vi "Test UI Manager API.vi"() -> ()   [LabVIEW 2022 SP3]
doc: "UI Manager API Tester.\n\n<b>Note:</b> This VI was modified by the <b>Validate DQMH Module</b> tool to add the 'Show Main VI Diagram on Init' functionality included in DQMH 6.1.\n\n<b>Note:</b> This VI was modified by the <b>Validate DQMH Module</b> tool to upgrade its Error Reported event frame to use an improved mechanism for displaying error information.\n\n____\nHAMPEL SOFTWARE ENGINEERING v2.6.0 (2023-12-19 10:54)"
uses:
  <vilib>/Utility/error.llb/DialogType.ctl
  <vilib>/Hampel Software Engineering/HSE Logger/LogRecord/LogRecord.lvclass/LogRecord.ctl
  UI Manager.lvlib
  Libraries/hse-libraries/Source/hse-dqmh/hse-dqmh.lvlib
  <vilib>/Hampel Software Engineering/HSE Logger/LogRecord/LogRecord.lvclass
  <vilib>/Hampel Software Engineering/HSE Logger/hse-logger.lvlib
panel:
  out "User Level":string
  out "User Name":string
  in  "Get User Level":bool
  in  "External Login":bool
  in  "Show Main VI Diagram on Init (F)":bool
  out "CLI Arguments out":string[](array[string])
  in  "Get CLI Arguments":bool
  in  "CLI Arguments in":string[](array[string])
  in  "Set CLI Arguments":bool
  in  "Remove Module from Run-Time Menu":bool
  in  "Descriptor":string
  in  "Shutdown Application":bool
  in  "Closeable?":bool
  in  "Set Window Closeable State":bool
  in  "Visible?":bool
  in  "Set Run-Time Menu Visibility":bool
  in  "Add Modules":bool
  in  "Modules Path":path
  in  "Add Mod to Menu":bool
  in  "Module DQMH Path":path
  in  "Btn_SystemMessage":bool
  in  "Prepare":bool
  in  "Configure":bool
  in  "Show PROJECT-ABOUT":bool
  in  "Show HSE-ABOUT":bool
  in  "Load RT Menu":bool
  in  "Run-Time Menu Path":path
  in  "Show Block Diagram":bool
  in  "Stop Module":bool
  in  "Start Module":bool
  in  "Hide Module Panel":bool
  in  "Show Module Panel":bool
  out "Status":string
  out "Module Running?":bool
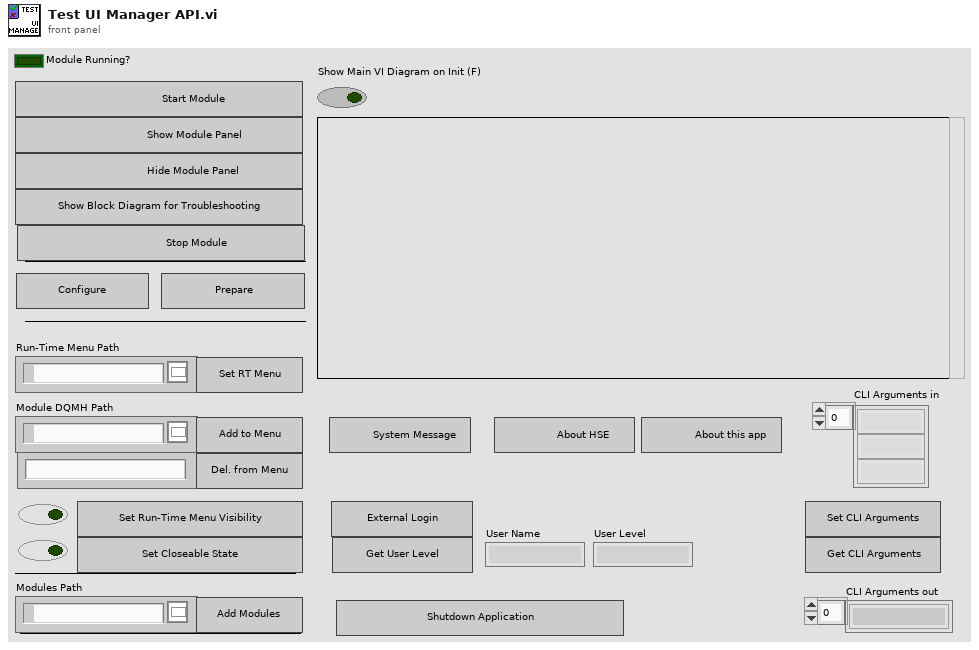
[diagram p1: front panel]
types:
  T1 = typedef "UI Manager.lvlib/Broadcast Events--cluster.ctl" = cluster{"Module Did Init":refnum<user-event>, "Status Updated":refnum<user-event>, "Error Reported":refnum<user-event>, "Module Did Stop":refnum<user-event>, "Update Module Execution Status":refnum<user-event>, "System Message":refnum<user-event>, "Login":refnum<user-event>, "Key down":refnum<user-event>}
  T2 = typedef "DialogType.ctl" = u16
  T3 = typedef "hse-dqmh.lvlib/System Message Source.ctl" = enum16{"module", "application", "network"}
  T4 = typedef "hse-logger.lvlib/LogLevel.ctl" = enum16{"DEBUG", "INFO", "WARNING", "ERROR", "CRITICAL"}
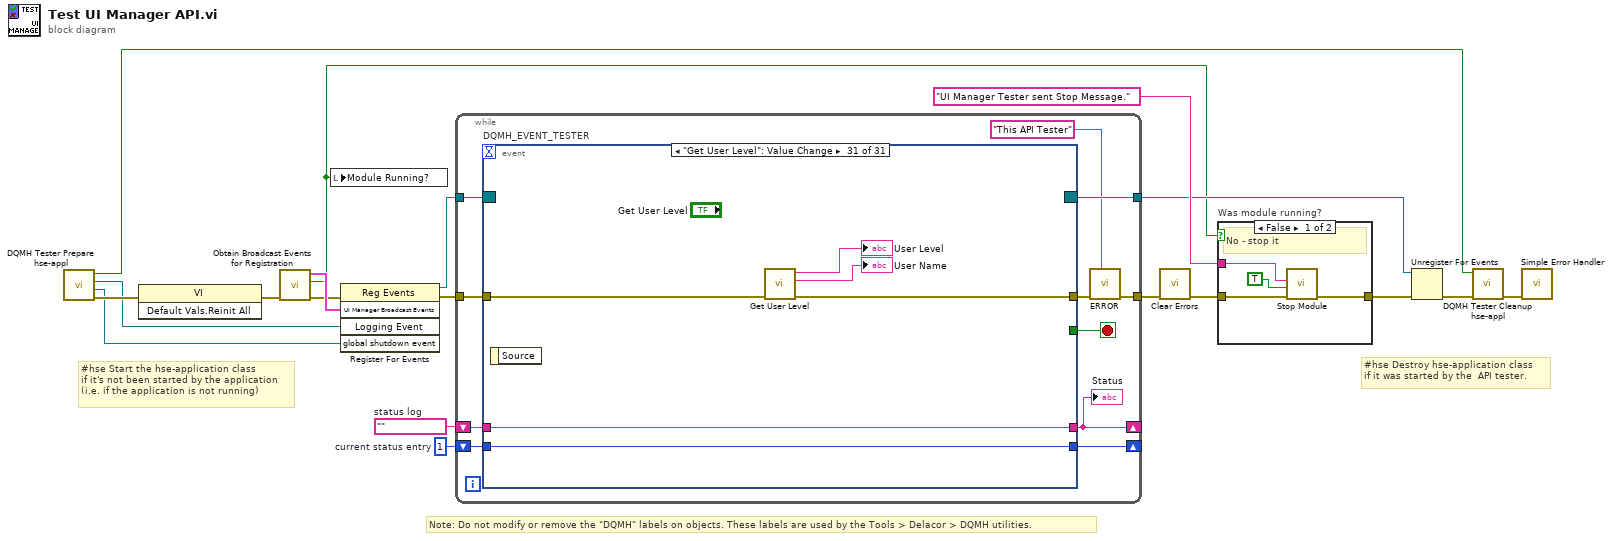
[diagram p0: block diagram]
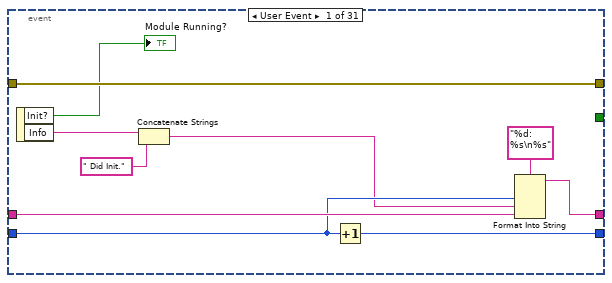
[diagram p3: hidden frame]
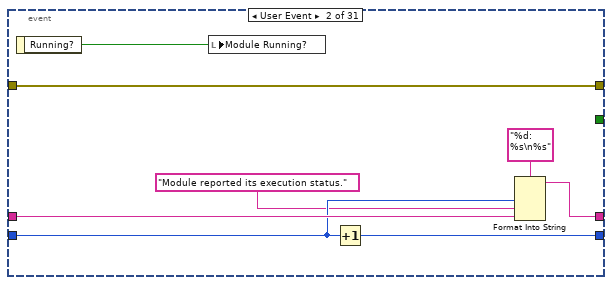
[diagram p4: hidden frame]
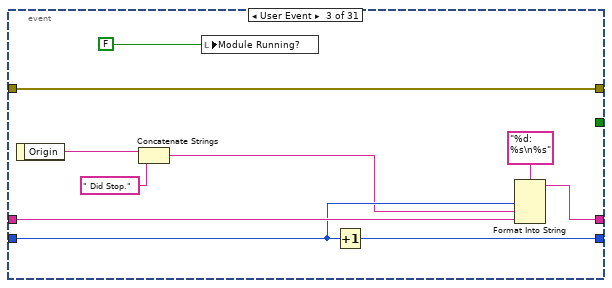
[diagram p5: hidden frame]
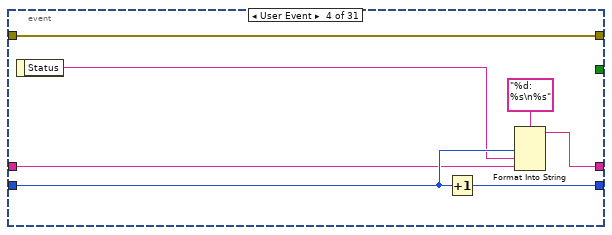
[diagram p6: hidden frame]
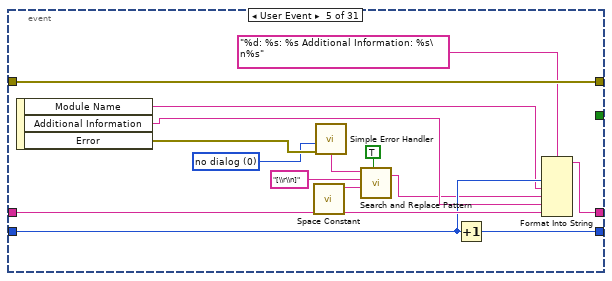
[diagram p7: hidden frame]
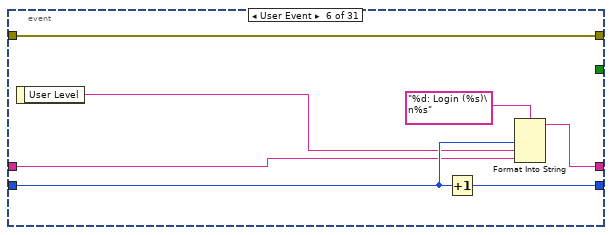
[diagram p8: hidden frame]
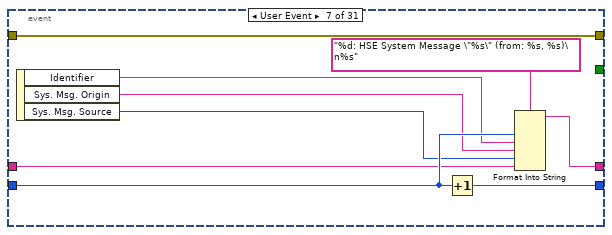
[diagram p9: hidden frame]
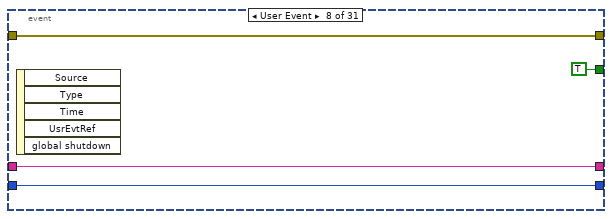
[diagram p10: hidden frame]
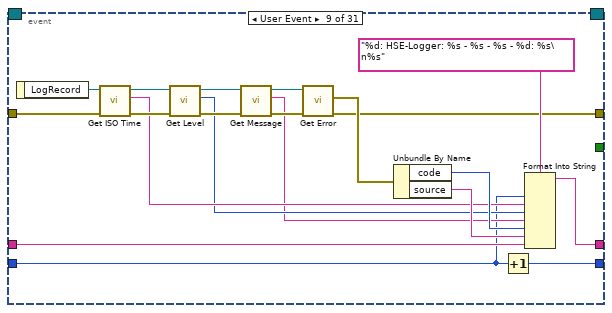
[diagram p11: hidden frame]
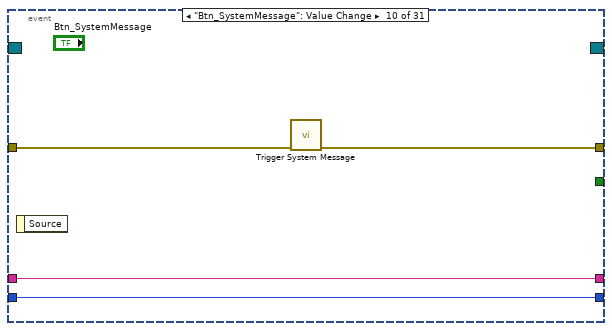
[diagram p12: hidden frame]
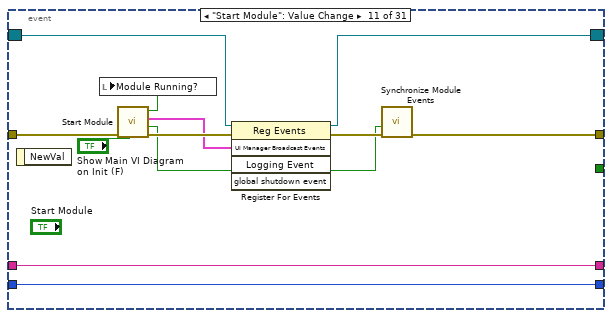
[diagram p13: hidden frame]
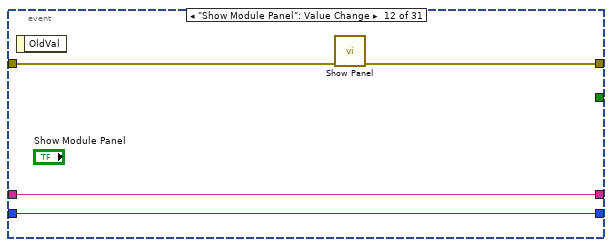
[diagram p14: hidden frame]
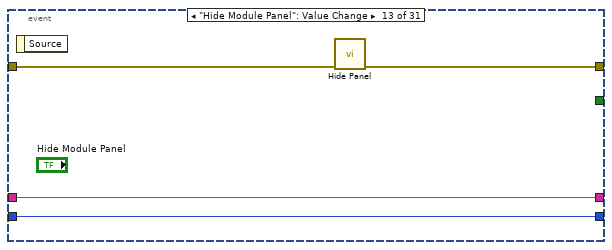
[diagram p15: hidden frame]
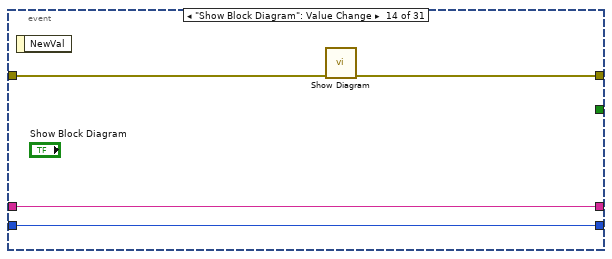
[diagram p16: hidden frame]
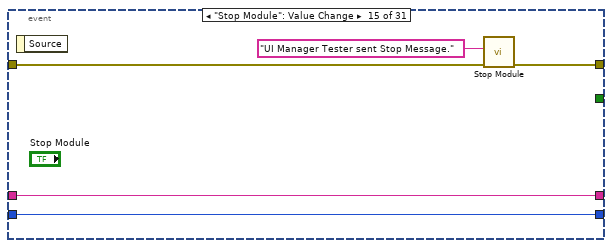
[diagram p17: hidden frame]
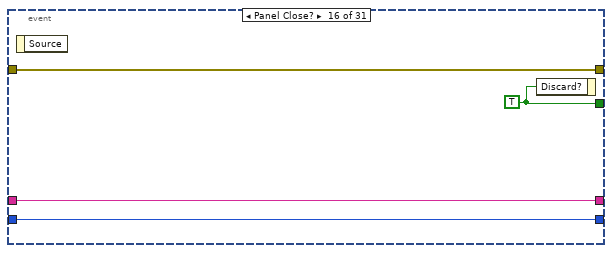
[diagram p18: hidden frame]
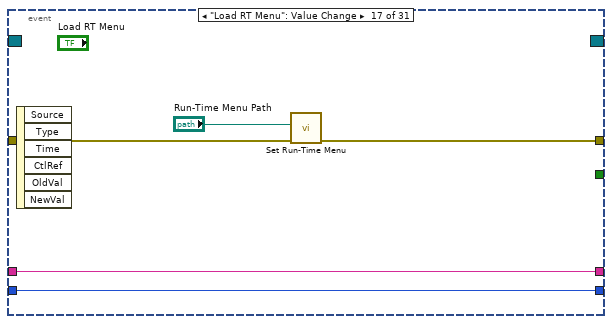
[diagram p19: hidden frame]
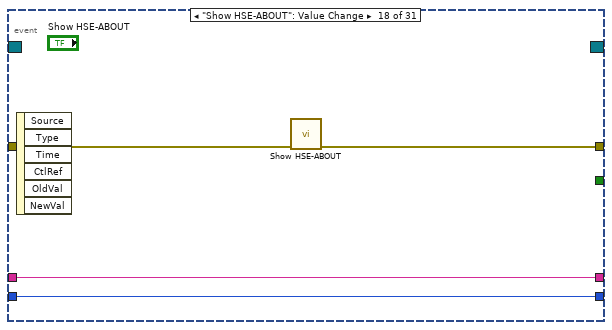
[diagram p20: hidden frame]
diagram:
  w16 = 1  # current status entry
  w17 = ""  # status log
  # "#hse Start the hse-application class \nif it's not been started by the application\n(i.e. if the application is not running)"
  # "#hse Destroy hse-application class \nif it was started by the  API tester."
  # "Note: Do not modify or remove the \"DQMH\" labels on objects. These labels are used by the Tools > Delacor > DQMH utilities."
  n1 = call "DQMH Tester Prepare hse-appl.vi"() -> ("error out"=w9:errorcluster, "global shutdown event"=w1:refnum<user-event>, "Logging Event"=w6:refnum<user-event>, "Started?"=w5:bool)  [unwired: 8 in]
  n2 = invoke class="VI" method="Default Vals.Reinit All"(error in=w9) -> (error out=w8:errorcluster)  [unwired: 2 in, 2 out]
  n3 = call "Obtain Broadcast Events for Registration.vi"("error in (no error)"=w8) -> ("error out"=w7:errorcluster, "Already running?"=w4:bool, "UI Manager Broadcast Events"=w14:T1)  [unwired: 8 in]
  n4 = local write "Module Running?"(w4) -> ()
  n5 = register-events(error in=w7, w14, w6, w1) -> (reference out=w13:refnum<event-registration>, error out=w15:errorcluster)  [unwired: 1 in]
  n6 = while {
    tunnel: w13 -> [w30]
    tunnel: [w21] -> w3
    shift-right: [w26] -> _
    shift-left: w17 -> [w28]
    shift-right: [w27] -> _
    shift-left: w16 -> [w29]
    tunnel: w15 -> [w25]
    tunnel: [w24] -> w12
    stop <- w22 stop-if-true
    n7 = event "DQMH_EVENT_TESTER" shown="[30] \"Get User Level\": Value Change" {
      selector: w30 -> [_ _ _ _ _ _ _ _ _ _ w129 _ _ _ _ _ _ _ _ _ _ _ _ _ _ _ _ _ _ _ _]
      dyn-events: [_ _ _ _ _ _ _ _ _ _ w128 _ _ _ _ _ _ _ _ _ _ _ _ _ _ _ _ _ _ _ _] -> w24
      timeout: _ -> [_ _ _ _ _ _ _ _ _ _ _ _ _ _ _ _ _ _ _ _ _ _ _ _ _ _ _ _ _ _ _]
      tunnel: [_ _ _ _ _ _ _ TRUE ("Discard?") _ _ _ _ _ _ _ w156 _ _ _ _ _ _ _ _ _ _ _ _ _ _ _] -> w22
      tunnel: [w40 w42 w49 w59 w80 w87 w95 w99 w102 w120 w127 w139 w143 w144 w150 w153 w158 w162 w166 w170 w174 w180 w186 w191 w196 w201 w206 w211 w216 w222 w228] -> w23
      tunnel: w29 -> [w36 w46 w56 w62 w77 w85 w93 w97 w103 w121 w132 w137 w141 w145 w151 w154 w159 w163 w167 w171 w175 w181 w187 w192 w197 w202 w207 w212 w217 w223 w229]
      tunnel: w28 -> [w37 w47 w57 w61 w79 w82 w89 w98 w104 w122 w133 w138 w142 w146 w152 w155 w160 w164 w168 w172 w176 w182 w188 w193 w198 w203 w208 w213 w218 w224 w230]
      tunnel: [w34 w44 w54 w63 w78 w83 w92 w98 w100 w122 w133 w138 w142 w146 w152 w155 w160 w164 w168 w172 w176 w182 w188 w193 w198 w203 w208 w213 w218 w224 w230] -> w26
      tunnel: [w35 w45 w55 w65 w76 w84 w93 w97 w101 w121 w132 w137 w141 w145 w151 w154 w159 w163 w167 w171 w175 w181 w187 w192 w197 w202 w207 w212 w217 w223 w229] -> w27
      tunnel: w25 -> [w40 w42 w49 w59 w80 w87 w95 w99 w105 w123 w126 w136 w140 w147 w148 w153 w161 w165 w169 w173 w177 w183 w189 w194 w199 w204 w209 w214 w219 w225 w231]
      event User Event {
        n8 = event-data() -> ("Init?"=→"Module Running?":bool, "Info"=w33:string)  [unwired: 1 in]
        n9 = Concatenate Strings(w33, " Did Init.") -> (w32:string)
        n10 = Increment(x=w36) -> (x+1=w35:i32)
        n11 = Format Into String(format string="%d: %s\n%s", w36, w32, w37) -> (resulting string=w34:string)  [unwired: 2 in, 1 out]
      }
      event User Event {
        n12 = event-data() -> ("Running?"=w41:bool)  [unwired: 1 in]
        n13 = local write "Module Running?"(w41) -> ()
        n14 = Increment(x=w46) -> (x+1=w45:i32)
        n15 = Format Into String(format string="%d: %s\n%s", w46, "Module reported its execution status.", w47) -> (resulting string=w44:string)  [unwired: 2 in, 1 out]
      }
      event User Event {
        n16 = event-data() -> ("Origin"=w53:string)  [unwired: 1 in]
        n17 = Concatenate Strings(w53, " Did Stop.") -> (w52:string)
        n18 = local write "Module Running?"(FALSE ("Module Did Init?")) -> ()
        n19 = Increment(x=w56) -> (x+1=w55:i32)
        n20 = Format Into String(format string="%d: %s\n%s", w56, w52, w57) -> (resulting string=w54:string)  [unwired: 2 in, 1 out]
      }
      event User Event {
        n21 = event-data() -> ("Status"=w60:string)  [unwired: 1 in]
        n22 = Increment(x=w62) -> (x+1=w65:i32)
        n23 = Format Into String(format string="%d: %s\n%s", w62, w60, w61) -> (resulting string=w63:string)  [unwired: 2 in, 1 out]
      }
      event User Event {
        w72 = T2 0 items=["no dialog", "OK message", "continue or stop message", "OK message + warnings", "continue/stop + warnings"] ("type of dialog (OK msg:1)")
        n24 = event-data() -> ("Module Name"=w73:string, "Additional Information"=w74:string, "Error"=w75:errorcluster)  [unwired: 1 in]
        n25 = call <vilib>:"Space Constant.vi"() -> ("String"=w68:string)
        n26 = call <vilib>:"Simple Error Handler.vi"("type of dialog (OK msg:1)"=w72, "error in (no error)"=w75) -> ("message"=w71:string)  [unwired: 3 in, 4 out]
        n27 = call <vilib>:"Search and Replace Pattern.vi"("string"=w71, "regular expression (\"\")"="[\\r\\n]" ("regular expression (\"\")"), "replace string (\"\")"=w68, "replace all? (F)"=TRUE ("replace all CR/LF with spaces")) -> ("result string"=w70:string)  [unwired: 1 in, 1 out]
        n28 = Increment(x=w77) -> (x+1=w76:i32)
        n29 = Format Into String(format string="%d: %s: %s Additional Information: %s\n%s", w77, w73, w70, w74, w79) -> (resulting string=w78:string)  [unwired: 2 in, 1 out]
      }
      event User Event {
        n30 = event-data() -> ("User Level"=w81:string)  [unwired: 1 in]
        n31 = Increment(x=w85) -> (x+1=w84:i32)
        n32 = Format Into String(format string="%d: Login (%s)\n%s", w85, w81, w82) -> (resulting string=w83:string)  [unwired: 2 in, 1 out]
      }
      event User Event {
        n33 = event-data() -> ("Identifier"=w91:string, "Sys. Msg. Origin"=w90:string, "Sys. Msg. Source"=w88:T3)  [unwired: 1 in]
        n34 = Increment(x=w93) -> ()  [unwired: 1 out]
        n35 = Format Into String(format string="%d: HSE System Message \"%s\" (from: %s, %s)\n%s", w93, w91, w90, w88, w89) -> (resulting string=w92:string)  [unwired: 2 in, 1 out]
      }
      event User Event {
        n36 = event-data() -> ()  [unwired: 1 in, 5 out]
      }
      event User Event {
        n37 = event-data() -> ("LogRecord"=w106:refnum<class "LogRecord.lvclass">)  [unwired: 1 in]
        n38 = call <vilib>:"Get ISO Time.vi"("error in"=w105, "LogRecord in"=w106) -> ("error out"=w119:errorcluster, "ISO Time"=w109:string, "LogRecord out"=w118:refnum<class "LogRecord.lvclass">)  [unwired: 7 in]
        n39 = call <vilib>:"Get Level.vi"("error in"=w119, "LogRecord in"=w118) -> ("error out"=w116:errorcluster, "Level"=w108:T4, "LogRecord out"=w117:refnum<class "LogRecord.lvclass">)  [unwired: 7 in]
        n40 = call <vilib>:"Get Message.vi"("error in"=w116, "LogRecord in"=w117) -> ("error out"=w114:errorcluster, "Message"=w107:string, "LogRecord out"=w115:refnum<class "LogRecord.lvclass">)  [unwired: 7 in]
        n41 = call <vilib>:"Get Error.vi"("error in"=w114, "LogRecord in"=w115) -> ("error out"=w102:errorcluster, "Error"=w110:errorcluster)  [unwired: 7 in, 1 out]
        n42 = Unbundle By Name(w110) -> ("code"=w112:i32, "source"=w111:string)
        n43 = Increment(x=w103) -> (x+1=w101:i32)
        n44 = Format Into String(format string="%d: HSE-Logger: %s - %s - %s - %d: %s\n%s", w103, w109, w108, w107, w112, w111, w104) -> (resulting string=w100:string)  [unwired: 2 in, 1 out]
      }
      event "Btn_SystemMessage": Value Change {
        n45 = event-data() -> ()  [unwired: 1 in, 1 out]
        n46 = call "Trigger System Message.vi"("error in (no error)"=w123) -> ("error out"=w120:errorcluster)  [unwired: 10 in]
      }
      event "Start Module": Value Change {
        n47 = event-data() -> ()  [unwired: 1 in, 1 out]
        n48 = call "Start Module.vi"("Show Main VI Diagram on Init (F)"="Show Main VI Diagram on Init (F)", "error in (no error)"=w126) -> ("error out"=w134:errorcluster, "Wait for Event Sync?"=w131:bool, "UI Manager Broadcast Events"=w130:T1, "Module Was Already Running?"=w125:bool)  [unwired: 6 in]
        n49 = local write "Module Running?"(w125) -> ()
        n50 = register-events(reference=w129, error in=w134, w130) -> (reference out=w128:refnum<event-registration>, error out=w135:errorcluster)  [unwired: 2 in]
        n51 = call "Synchronize Module Events.vi"("error in (no error)"=w135, "Wait for Event Sync?"=w131) -> ("error out"=w127:errorcluster)  [unwired: 9 in]
      }
      event "Show Module Panel": Value Change {
        n52 = event-data() -> ()  [unwired: 1 in, 1 out]
        n53 = call "Show Panel.vi"("error in (no error)"=w136) -> ("error out"=w139:errorcluster)  [unwired: 10 in]
      }
      event "Hide Module Panel": Value Change {
        n54 = event-data() -> ()  [unwired: 1 in, 1 out]
        n55 = call "Hide Panel.vi"("error in (no error)"=w140) -> ("error out"=w143:errorcluster)  [unwired: 10 in]
      }
      event "Show Block Diagram": Value Change {
        n56 = event-data() -> ()  [unwired: 1 in, 1 out]
        n57 = call "Show Diagram.vi"("error in (no error)"=w147) -> ("error out"=w144:errorcluster)  [unwired: 10 in]
      }
      event "Stop Module": Value Change {
        n58 = event-data() -> ()  [unwired: 1 in, 1 out]
        n59 = call "Stop Module.vi"("error in (no error)"=w148, "Origin"="UI Manager Tester sent Stop Message.") -> ("error out"=w150:errorcluster)  [unwired: 9 in]
      }
      event Panel Close? {
        w156 = TRUE ("Discard?")
        n60 = event-data() -> ()  [unwired: 1 in, 1 out]
        n61 = event-data("Discard?"=w156) -> ()  [unwired: 1 in, 1 out]
      }
      event "Load RT Menu": Value Change {
        n62 = event-data() -> ()  [unwired: 1 in, 6 out]
        n63 = call "Set Run-Time Menu.vi"("error in (no error)"=w161, "Run-Time Menu Path"="Run-Time Menu Path") -> ("error out"=w158:errorcluster)  [unwired: 9 in]
      }
      event "Show HSE-ABOUT": Value Change {
        n64 = event-data() -> ()  [unwired: 1 in, 6 out]
        n65 = call "Show HSE-ABOUT.vi"("error in (no error)"=w165) -> ("error out"=w162:errorcluster)  [unwired: 10 in]
      }
      event "Show PROJECT-ABOUT": Value Change {
        n66 = event-data() -> ()  [unwired: 1 in, 6 out]
        n67 = call "Show PROJECT-ABOUT.vi"("error in (no error)"=w169) -> ("error out"=w166:errorcluster)  [unwired: 10 in]
      }
      event "Configure": Value Change {
        n68 = event-data() -> ()  [unwired: 1 in, 6 out]
        n69 = call "Configure.vi"("error in (no error)"=w173) -> ("error out"=w170:errorcluster)  [unwired: 10 in]
      }
      event "Prepare": Value Change {
        n70 = event-data() -> ()  [unwired: 1 in, 6 out]
        n71 = call "Prepare.vi"("error in (no error)"=w177) -> ("error out"=w174:errorcluster)  [unwired: 10 in]
      }
      event "Add Mod to Menu": Value Change {
        n72 = event-data() -> ()  [unwired: 1 in, 1 out]
        n73 = call "Add Module to Run-Time Menu.vi"("error in (no error)"=w183, "Module Descriptor"="Descriptor", "Module DQMH Path"="Module DQMH Path") -> ("error out"=w180:errorcluster)  [unwired: 8 in]
      }
      event "Add Modules": Value Change {
        n74 = event-data() -> ()  [unwired: 1 in, 1 out]
        n75 = Build Array("Modules Path") -> (w184:path[])
        n76 = call "Set Modules.vi"("error in (no error)"=w189, "Module Paths"=w184) -> ("error out"=w186:errorcluster)  [unwired: 8 in, 1 out]
      }
      event "Set Run-Time Menu Visibility": Value Change {
        n77 = event-data() -> ()  [unwired: 1 in, 1 out]
        n78 = call "Set Run-Time Menu Visibility.vi"("error in (no error)"=w194, "Visible?"="Visible?") -> ("error out"=w191:errorcluster)  [unwired: 9 in]
      }
      event "Set Window Closeable State": Value Change {
        n79 = event-data() -> ()  [unwired: 1 in, 6 out]
        n80 = call "Set Window Closeable State.vi"("error in (no error)"=w199, "Closeable?"="Closeable?") -> ("error out"=w196:errorcluster)  [unwired: 9 in]
      }
      event "Shutdown Application": Value Change {
        w200 = TRUE  # User Confirm?
        # "#CodeNeeded\n1. Position the new \"Test Shutdown Application\" button appropriately on the front panel.\n2. Delete or edit this label when done."
        n81 = event-data() -> ()  [unwired: 1 in, 1 out]
        n82 = call "Shutdown Application.vi"("error in (no error)"=w204, "User Confirm?"=w200) -> ("error out"=w201:errorcluster)  [unwired: 9 in]
      }
      event "Remove Module from Run-Time Menu": Value Change {
        n83 = event-data() -> ()  [unwired: 1 in, 1 out]
        n84 = local read "Module DQMH Path"() -> (w205:path)
        n85 = call "Remove Module from Run-Time Menu.vi"("error in (no error)"=w209, "Module DQMH Path"=w205) -> ("error out"=w206:errorcluster)  [unwired: 9 in]
      }
      event "Set CLI Arguments": Value Change {
        n86 = event-data() -> ()  [unwired: 1 in, 1 out]
        n87 = call "Set CLI Arguments.vi"("error in"=w214, "CLI Arguments"="CLI Arguments in") -> ("error out"=w211:errorcluster)  [unwired: 8 in, 1 out]
      }
      event "Get CLI Arguments": Value Change {
        n88 = event-data() -> ()  [unwired: 1 in, 1 out]
        n89 = call "Get CLI Arguments.vi"("error in"=w219) -> ("error out"=w216:errorcluster, "CLI Arguments"=→"CLI Arguments out":string[])  [unwired: 8 in, 1 out]
      }
      event "External Login": Value Change {
        w220 = "operator"  # User Level
        w221 = "Adam"  # User Name
        n90 = event-data() -> ()  [unwired: 1 in, 1 out]
        n91 = call "External Login.vi"("error in"=w225, "User Name"=w221, "User Level"=w220) -> ("error out"=w222:errorcluster)  [unwired: 8 in]
      }
      event "Get User Level": Value Change {
        n92 = event-data() -> ()  [unwired: 1 in, 1 out]
        n93 = call "Get User Level.vi"("error in"=w231) -> ("error out"=w228:errorcluster, "User Name"=→"User Name":string, "User Level"=→"User Level":string)  [unwired: 7 in, 1 out]
      }
    }
    "Status" <- w26
    n94 = call <vilib>:"ERROR.vi"("Message"="This API Tester" ("Origin"), "error in"=w23) -> ("error out"=w21:errorcluster)  [unwired: 9 in]
  }
  n95 = call <vilib>:"Clear Errors.vi"("error in (no error)"=w3) -> ("error out"=w11:errorcluster)  [unwired: 5 in, 1 out]
  n96 = case "Was module running?" shown="False" w4 {
    tunnel: [w235 w236] -> w19
    tunnel: "UI Manager Tester sent Stop Message." ("Origin") -> [w232 _]
    tunnel: w11 -> [w233 w236]
    frame False {
      # "No - stop it"
      n97 = call "Stop Module.vi"("error in (no error)"=w233, "Wait for Module to Stop? (F)"=TRUE ("Wait for Module to stop?"), "Origin"=w232) -> ("error out"=w235:errorcluster)  [unwired: 8 in]
    }
    frame True {
      # "yes - do nothing"
    }
  }
  n98 = Unregister For Events(event registration refnum=w12, error in=w19) -> (error out=w10:errorcluster)
  n99 = call "DQMH Tester Cleanup hse-appl.vi"("error in"=w10, "Stop?"=w5) -> ("error out"=w2:errorcluster)  [unwired: 9 in]
  n100 = call <vilib>:"Simple Error Handler.vi"("error in (no error)"=w2) -> ()  [unwired: 4 in, 5 out]
